vi "HTTP.Read Request Headers.vi"(8 "error in (no error)":errorcluster, 11 "Connection.WS in":refnum<class "Connection.WS.lvclass">) -> (0 "error out":errorcluster, 3 "Connection.WS out":refnum<class "Connection.WS.lvclass">)   [LabVIEW 2013, in "Connection.WS_GOSPL.lvlib" / "Connection.WS.lvclass"]
uses:
  Connection.WS.lvclass
  Connection/Connection.lvclass/Connection.ctl
  Connection.WS.lvclass/Connection.WS.ctl
  Connection/Connection.lvclass
  Connection.TCP/Connection.TCP.lvclass
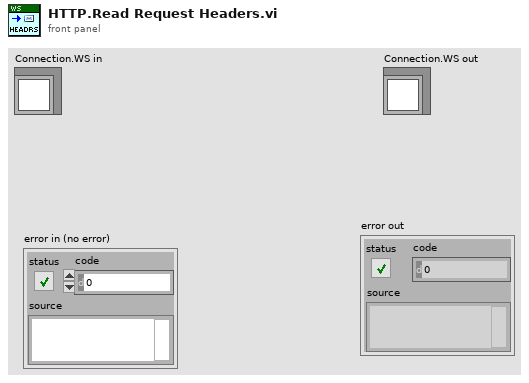
[diagram p1: front panel]
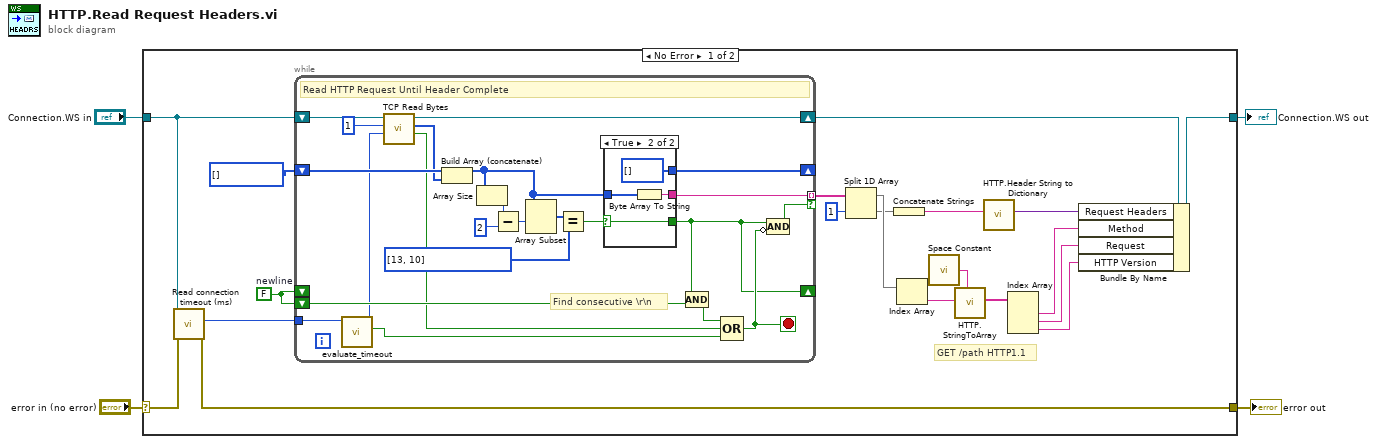
[diagram p0: block diagram]
diagram:
  n1 = case shown="No Error" "error in (no error)" {
    selector: "error in (no error)" -> [w14 w54]
    tunnel: "Connection.WS in" -> [w24 w55]
    tunnel: [w5 w55] -> w3
    tunnel: [w13 w54] -> w1
    frame No Error {
      w23 = FALSE  # newline
      # "GET /path HTTP1.1"
      n2 = call "Read connection timeout (ms).vi"("error in (no error)"=w14, "Connection in"=w24) -> ("error out"=w13:errorcluster, "connection timeout (ms)"=w15:i32)  [unwired: 7 in, 1 out]
      n3 = while {
        tunnel: w15 -> [w47]
        shift-right: [w40] -> w6
        shift-left: w24 -> [w42]
        shift-right: [w34] -> _
        shift-left: u8[] [] ("element") -> [w46]
        shift-right: [w30] -> _
        shift-left: w23 -> [_]
        tunnel: [w32] -> w18 mode=indexing if=w36
        shift-left: w23 -> [w33]
        stop <- w37 stop-if-true
        # "Find consecutive \\r\\n"
        # "Read HTTP Request Until Header Complete"
        n4 = call "evaluate_timeout.vi"("timeout (ms)"=w47) -> ("elapsed"=w26:bool, "remaining timeout (ms)"=w27:i32)  [unwired: 9 in]
        n5 = call "TCP Read Bytes.vi"("timeout (1000 ms)"=w27, "bytes to read (100)"=1, "Connection.TCP"=w42) -> ("timed out"=w25:bool, "Bytes"=w39:u8[], "Connection.TCP"=w40:refnum<class "Connection.WS.lvclass">)  [unwired: 4 in, 2 out]
        n6 = Build Array (concatenate)(w46, w39) -> (w35:u8[])
        n7 = Array Size(array=w35) -> (size(s)=w45:i32)
        n8 = Subtract(x=w45, y=2 ("length")) -> (x-y=w43:i32)
        n9 = Array Subset(array=w35, index=w43) -> (w38:u8[])  [unwired: 1 in]
        n10 = Equal?(x=w38, y=u8[] [13, 10] ("element")) -> (x = y?=w31:bool)
        n11 = case shown="True" w31 {
          selector: w31 -> [w48 w50]
          tunnel: w35 -> [w49 w51]
          tunnel: [w49 u8[] [] ("element")] -> w34
          tunnel: [_ w52] -> w32
          tunnel: [w48 w50] -> w30
          frame False {
          }
          frame True {
            n12 = Byte Array To String(unsigned byte array=w51) -> (string=w52:string)
          }
        }
        n13 = Compound Arithmetic op=AND(w30, w33) -> (w29:bool)
        n14 = Compound Arithmetic op=OR(w29, w25, w26) -> (w37:bool)
        n15 = Compound Arithmetic op=AND(w30, invert w37) -> (w36:bool)
      }
      n16 = Split 1D Array(array=w18, index=1) -> (first subarray=w22:string[], second subarray=w20:string[])
      n17 = Concatenate Strings(w20) -> (w21:string)
      n18 = Index Array(array=w22) -> (element=w12:string)  [unwired: 1 in]
      n19 = call <vilib>:"Space Constant.vi"() -> ("String"=w7:string)
      n20 = call "HTTP.StringToArray.vi"("Separator"=w7, "string"=w12) -> ("Array"=w8:string[])  [unwired: 9 in]
      n21 = call "HTTP.Header String to Dictionary.vi"("HTTP Header"=w21) -> ("Dictionary"=w17:variant)  [unwired: 10 in]
      n22 = Index Array(array=w8) -> (element #1=w11:string, element #2=w10:string, element #3=w9:string)  [unwired: 3 in]
      n23 = Bundle By Name(cluster=w6, "Request Headers"=w17, "Method"=w11, "Request"=w10, "HTTP Version"=w9) -> (w5:refnum<class "Connection.WS.lvclass">)
    }
    frame Error {
    }
  }
  "Connection.WS out" <- w3
  "error out" <- w1
